vi "Sgl_ReadAttribute.vi"(5 "error in (no error)":errorcluster) -> (19 "error out":errorcluster)   [LabVIEW 2016]
uses:
  <resource>/Framework/Providers/Open_GDS/ClassProviders/Provider_EndevoGOOP300/Templates/SingletonTemplate/SingletonTemplate.lvclass
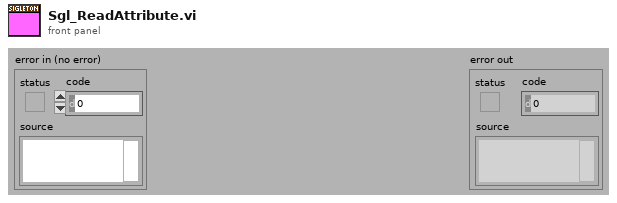
[diagram p1: front panel]
types:
  T1 = typedef "SingletonTemplate.lvclass/ObjectAttributes.ctl" = cluster{"Attribute1":dbl}
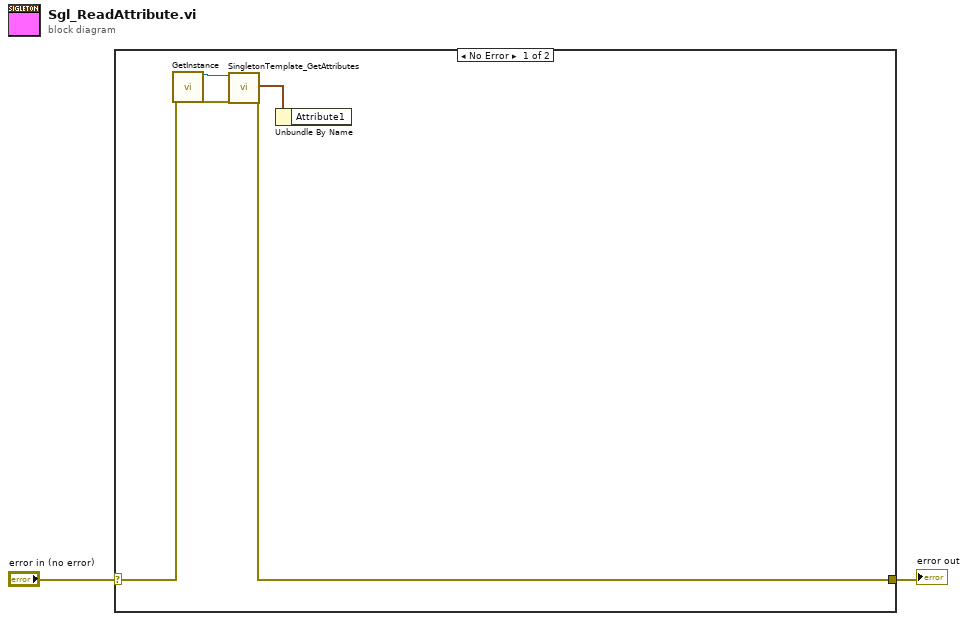
[diagram p0: block diagram]
diagram:
  n1 = case shown="No Error" "error in (no error)" {
    selector: "error in (no error)" -> [w3 w8]
    tunnel: [w6 w8] -> w1
    frame No Error {
      n2 = call <resource>:"GetInstance.vi"("error in (no error)"=w3) -> ("reference out"=w4:refnum<class "SingletonTemplate.lvclass">, "error out"=w5:errorcluster)  [unwired: 17 in]
      n3 = call <resource>:"SingletonTemplate_GetAttributes.vi"("reference in"=w4, "error in (no error)"=w5) -> ("Attributes"=w7:T1, "error out"=w6:errorcluster)  [unwired: 14 in, 2 out]
      n4 = Unbundle By Name(w7) -> ()  [unwired: 1 out]
    }
    frame Error {
    }
  }
  "error out" <- w1
